vi "Leds.vi"(3 "Message":string) -> (0 "Boolean":bool, 1 "number":i32)   [LabVIEW 2019]
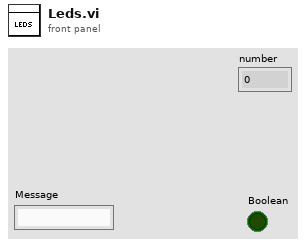
[diagram p1: front panel]
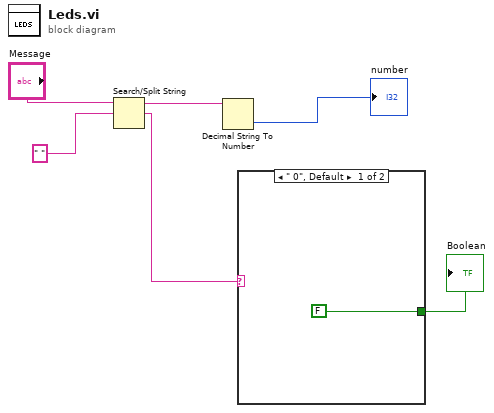
[diagram p0: block diagram]
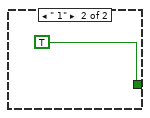
[diagram p2: hidden frame]
diagram:
  n1 = Search/Split String(string="Message", search string/char (-)=" ") -> (substring before match=w4:string, match + rest of string=w1:string)  [unwired: 1 in, 1 out]
  n2 = Decimal String To Number(string=w4) -> (number=→"number":i32)  [unwired: 2 in, 1 out]
  n3 = case shown="\" 0\", Default" w1 {
    tunnel: [FALSE TRUE] -> w2
    frame " 0", Default {
    }
    frame " 1" {
    }
  }
  "Boolean" <- w2
